vi "Find Workspace.vi"(8 "error in (no error)":errorcluster, 10 "Control In":T2, 11 "Component.lvclass":refnum<class "Component Tray.lvclass">) -> (0 "error out":errorcluster, 1 "Workspace":T1, 2 "Control Out":T2, 3 "Workspace Out":refnum<class "Component Tray.lvclass">)   [LabVIEW 2020, in "Component Tray.lvclass"]
uses:
  Component Tray.lvclass
  Controller/Controllers.ctl
  Controller/I-O/I-O.lvclass
  Controller/Dispenser/Dispenser.lvclass
  C:/Program Files (x86)/Aerotech/A3200/LabVIEW/2010/Bin/Aerotech.A3200.dll
  Program Files (x86)/Aerotech/A3200/LabVIEW/2010/Bin/Aerotech.A3200.dll
  Workspace.ctl
  C:/Users/hep/Documents/CMU gantry/Classes/Workspace/Fixture.lvclass
  Fixture.lvclass/Fixture.ctl
  Read Fixture ID.vi
  Read Position.vi
  Fixture.lvclass
  Controller/Controller.lvclass
panel:
  out "XYZTheta":dbl[](array[numeric]) format="%#.6g"
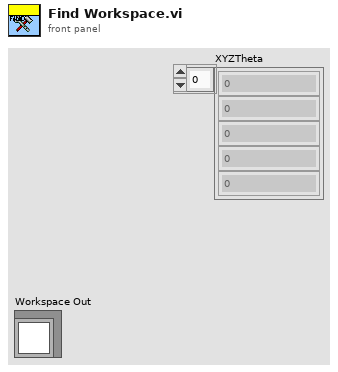
[diagram p1: front panel]
types:
  T1 = typedef "Fixture.lvclass/Workspace.ctl" = cluster{"XYZTheta":dbl[], "Workspace Valve":i32, "Workspace Sensor":i32}
  T2 = typedef "Controller.lvclass/Controllers.ctl" = cluster{"I-O.lvclass":refnum<class "I-O.lvclass">, "Dispenser.lvclass":refnum<class "Dispenser.lvclass">, "Gantry":refnum<k24>}
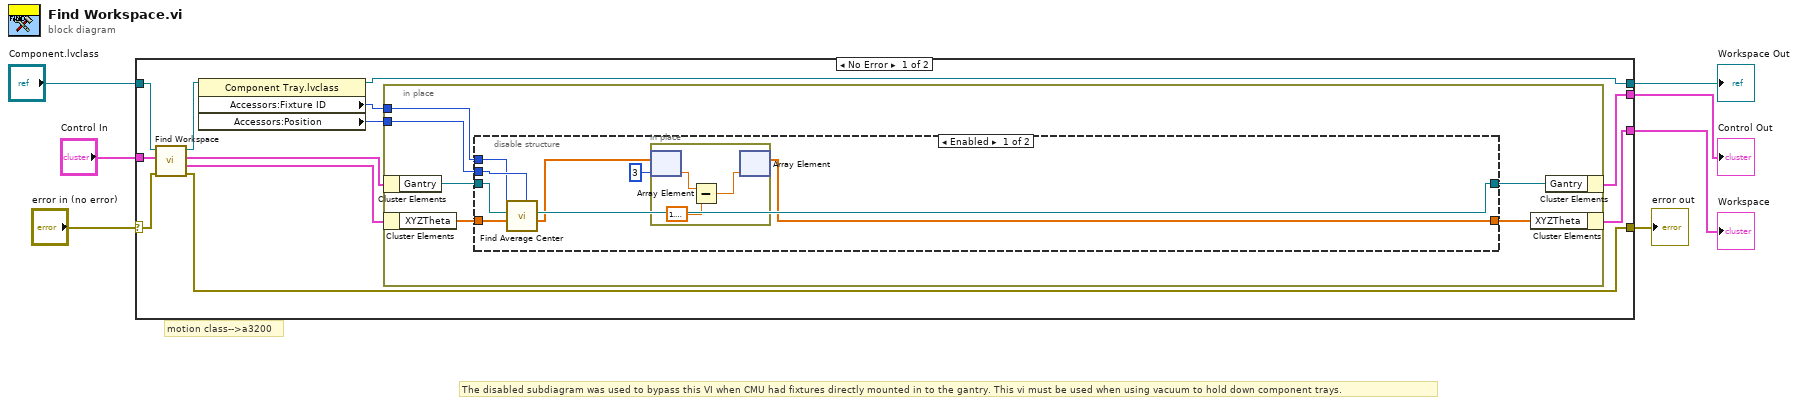
[diagram p0: block diagram]
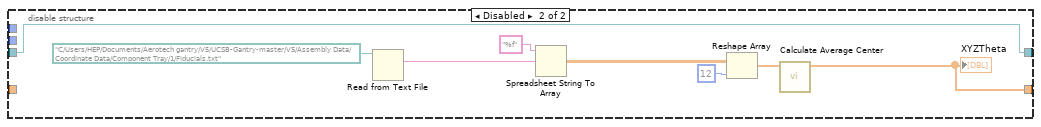
[diagram p2: hidden frame]
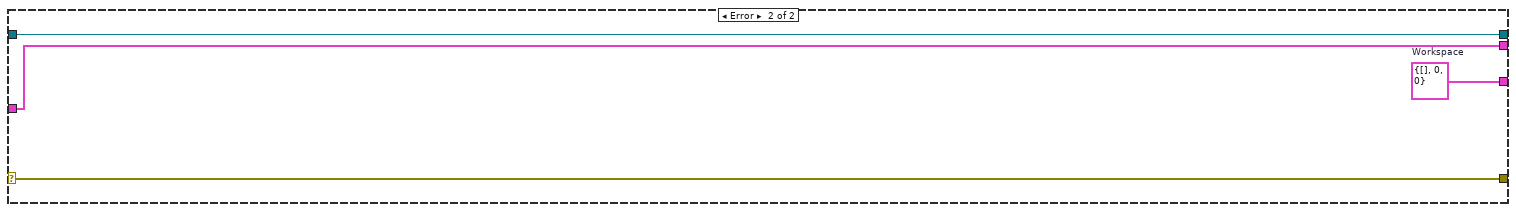
[diagram p3: hidden frame]
diagram:
  # "The disabled subdiagram was used to bypass this VI when CMU had fixtures directly mounted in to the gantry. This vi must be used when using vacuum to hold down component trays."
  # "motion class-->a3200"
  n1 = case shown="No Error" "error in (no error)" {
    selector: "error in (no error)" -> [w17 w48]
    tunnel: [w13 w47] -> w7
    tunnel: [w19 w48] -> w6
    tunnel: [w12 w46] -> w5
    tunnel: "Control In" -> [w16 w47]
    tunnel: [w8 w45] -> w2
    tunnel: "Component.lvclass" -> [w15 w45]
    frame No Error {
      n2 = call-parent "Find Workspace.vi"("Error In"=w17, "Control In"=w16, "Workspace In"=w15) -> ("Error Out"=w19:errorcluster, 1:"Workspace Out"=w18:T1, "Control Out"=w14:T2, 3:"Workspace Out"=w9:refnum<class "Component Tray.lvclass">)  [unwired: 5 in]
      n3 = property class="Component Tray.lvclass"(reference=w9) -> (reference out=w8:refnum<class "Component Tray.lvclass">, "Accessors:Fixture ID"=w11:i32, "Accessors:Position"=w10:i32)  [unwired: 1 in, 1 out]
      n4 = in-place {
        in-place-border: w11 -> [w24]
        in-place-border: w10 -> [w25]
        n5 = in-place-cluster #1(w14) -> ("Gantry"=w23:refnum<k24>)
        n6 = in-place-cluster #2(w18) -> ("XYZTheta"=w22:dbl[])
        n7 = disable-structure shown="Enabled" {
          disable-tunnel: w25 -> [w30 _]
          disable-tunnel: w24 -> [w29 _]
          disable-tunnel: w23 -> [w33 w37]
          disable-tunnel: w22 -> [w32 _]
          disable-tunnel: [w26 w38] -> w21
          disable-tunnel: [w31 w37] -> w20
          frame Enabled {
            n8 = call "Find Average Center.vi"("Position"=w30, "Tray Number"=w29, "XYZTheta"=w32, "Gantry 2"=w33) -> ("XYZTheta"=w28:dbl[], "Gantry 3"=w31:refnum<k24>)  [unwired: 4 in]
            n9 = in-place {
              n10 = in-place-array #3(w28, 3) -> (w36:dbl)
              n11 = Subtract(x=w36, y=1.5707963267948966) -> (x-y=w34:dbl)
              n12 = in-place-array #3(w34) -> (w26:dbl[])  [unwired: 1 out]
            }
          }
          frame Disabled {
            n13 = Read from Text File(file (use dialog)=path "C:/Users/HEP/Documents/Aerotech gantry/V5/UCSB-Gantry-master/V5/Assembly Data/Coordinate Data/Component Tray/1/Fiducials.txt") -> (text=w42:string)  [unwired: 3 in, 3 out]
            n14 = Spreadsheet String To Array(format string="%f", spreadsheet string=w42) -> (array=w41:dbl[][])  [unwired: 2 in]
            n15 = Reshape Array(w41, 12 ("dimension size")) -> (w39:dbl[])
            n16 = call "Calculate Average Center.vi"("Gantry Fiducials"=w39) -> ("XYZTheta"=w38:dbl[])  [unwired: 10 in]
            "XYZTheta" <- w38
          }
        }
        n17 = in-place-cluster #2("XYZTheta"=w21) -> (w12:T1)
        n18 = in-place-cluster #1("Gantry"=w20) -> (w13:T2)
      }
    }
    frame Error {
      w46 = T1 {"XYZTheta"=[], "Workspace Valve"=0, "Workspace Sensor"=0}  # Workspace
    }
  }
  "error out" <- w6
  "Control Out" <- w7
  "Workspace" <- w5
  "Workspace Out" <- w2
